vi "Flatten.vi"(8 "error in":errorcluster, 9 "Data":T1) -> (0 "error out":errorcluster, 2 "Buffer":u8[](array[numeric]) format="%.0x")   [LabVIEW 2020, in "DoubleData.lvlib"]
uses:
  DoubleData.lvlib
  Data.ctl
  lv-protoc/LV-Proto/LV-Proto.lvlib
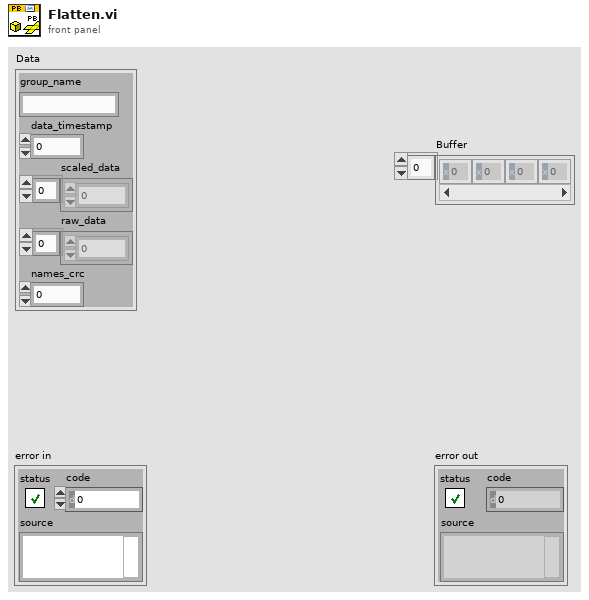
[diagram p1: front panel]
types:
  T1 = typedef "DoubleData.lvlib/Data.ctl" = cluster{"group_name":string, "data_timestamp":i64, "scaled_data":dbl[], "raw_data":dbl[], "names_crc":u32}
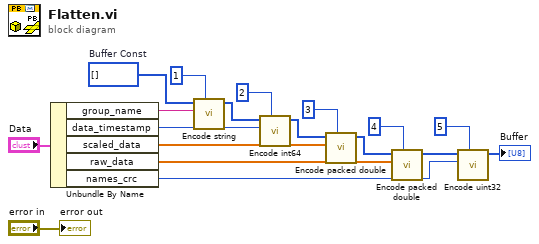
[diagram p0: block diagram]
diagram:
  w16 = u8[] []  # Buffer Const
  n1 = Unbundle By Name("Data") -> ("group_name"=w14:string, "data_timestamp"=w11:i64, "scaled_data"=w8:dbl[], "raw_data"=w5:dbl[], "names_crc"=w2:u32)
  n2 = call "Encode string.vi"("Field Number"=1, "string"=w14, "Buffer in"=w16) -> ("Buffer"=w13:u8[])  [unwired: 8 in]
  n3 = call "Encode int64.vi"("Field Number"=2, "int64"=w11, "Buffer in"=w13) -> ("Buffer"=w10:u8[])  [unwired: 8 in]
  n4 = call "Encode packed double.vi"("Field Number"=3, "double"=w8, "Buffer in"=w10) -> ("Buffer"=w7:u8[])  [unwired: 8 in]
  n5 = call "Encode packed double.vi"("Field Number"=4, "double"=w5, "Buffer in"=w7) -> ("Buffer"=w4:u8[])  [unwired: 8 in]
  n6 = call "Encode uint32.vi"("Field Number"=5, "uint32"=w2, "Buffer in"=w4) -> ("Buffer"=→"Buffer":u8[])  [unwired: 8 in]
  "error out" <- "error in"
